vi "Read quoted string.vi"(11 "StringFormatter in":refnum<class "StringFormatter.lvclass">) -> (2 "quoted string":bool, 3 "StringFormatter out":refnum<class "StringFormatter.lvclass">)   [LabVIEW 2013, in "OpenStringFormatter.lvlib" / "StringFormatter.lvclass"]
uses:
  StringFormatter.lvclass
  StringFormatter.lvclass/StringFormatter.ctl
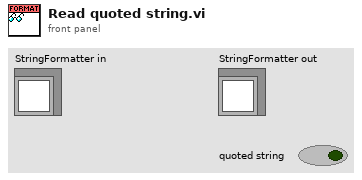
[diagram p1: front panel]
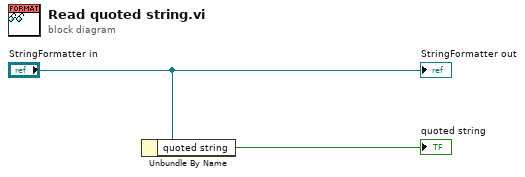
[diagram p0: block diagram]
diagram:
  n1 = Unbundle By Name("StringFormatter in") -> ("quoted string"=→"quoted string":bool)
  "StringFormatter out" <- "StringFormatter in"
